vi "Fetch Waveform.vi"(8 "error in (no error)":errorcluster, 10 "Channel":string, 11 "Thermometer DAQmx Base CFG in":refnum<class "Thermometer DAQmx Base CFG.lvclass">) -> (0 "error out":errorcluster, 2 "Waveform":waveform(dbl), 3 "Thermometer DAQmx Base CFG out":refnum<class "Thermometer DAQmx Base CFG.lvclass">)   [LabVIEW 2023, in "Thermometer DAQmx Base CFG.lvclass"]
uses:
  Thermometer DAQmx Base CFG.lvclass
  DAQmx/DAQmx Base CFG/DAQmx Base CFG.lvclass/DAQmx Base CFG.ctl
  Thermometer DAQmx Base CFG.lvclass/Thermometer DAQmx Base CFG.ctl
  <vilib>/DAQmx/read.llb/DAQmx Read (Analog 1D Wfm NChan NSamp).vi
  <vilib>/Waveform/WDTOps.llb/WDT Append Waveforms DBL.vi
  <vilib>/DAQmx/miscellaneous.llb/DAQmx Fill In Error Info.vi
  <vilib>/Utility/error.llb/Error Cluster From Error Code.vi
  <vilib>/ErrorRing/Error Ring.xnode
  <resource>/objmgr/daqmx.rc
  DAQmx/DAQmx Base CFG/DAQmx Base CFG.lvclass
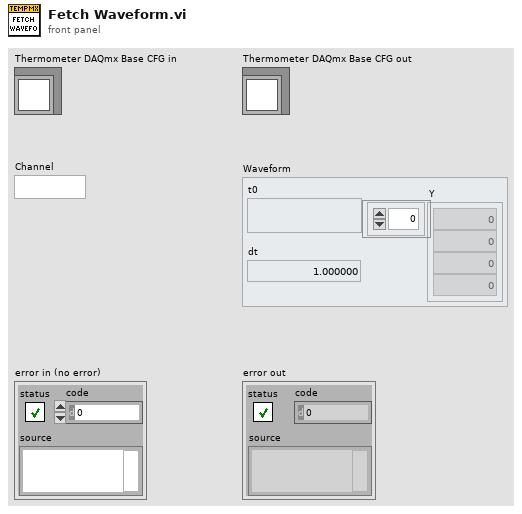
[diagram p1: front panel]
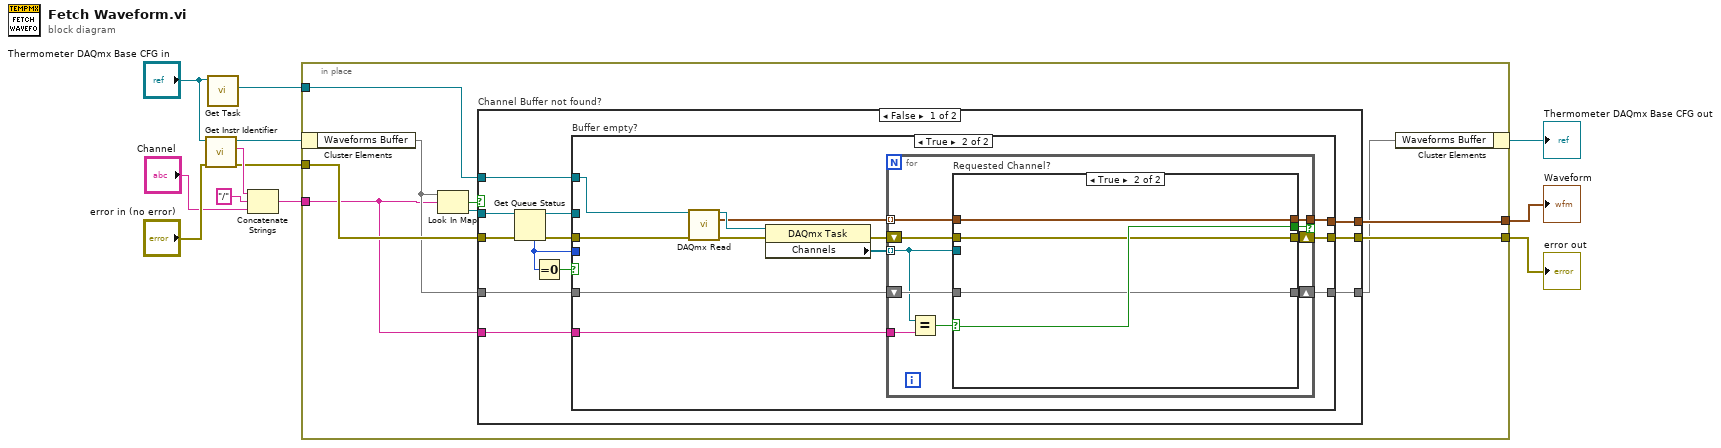
[diagram p0: block diagram]
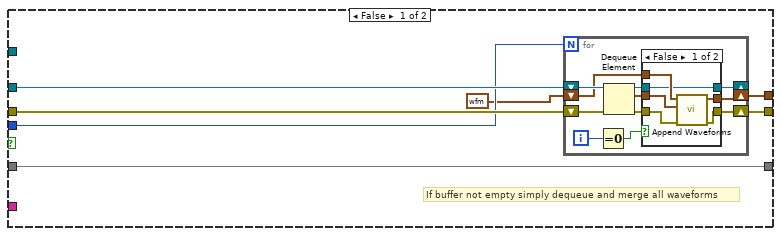
[diagram p2: hidden frame]
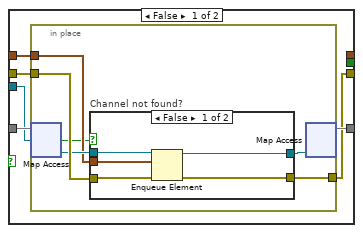
[diagram p4: hidden frame]
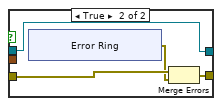
[diagram p5: hidden frame]
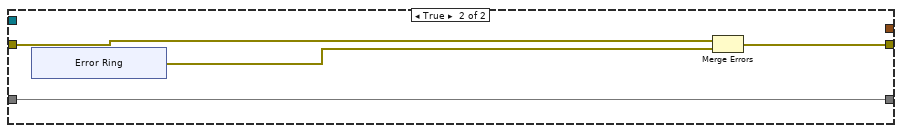
[diagram p6: hidden frame]
diagram:
  n1 = call-dynamic "Get Instr Identifier.vi"("error in (no error)"="error in (no error)", "Configuration Base in"="Thermometer DAQmx Base CFG in") -> ("error out"=w6:errorcluster, "Instr Ident"=w11:string, "Configuration Base out"=w8:refnum<class "Thermometer DAQmx Base CFG.lvclass">)  [unwired: 7 in]
  n2 = call "Get Task.vi"("DAQmx Base CFG in"="Thermometer DAQmx Base CFG in") -> ("Task"=w1:refnum<k21>)  [unwired: 9 in, 1 out]
  n3 = Concatenate Strings(w11, "/" ("string"), "Channel") -> (w7:string)
  n4 = in-place {
    in-place-border: w7 -> [w17]
    in-place-border: w6 -> [w21]
    in-place-border: [w20] -> w5
    in-place-border: [w19] -> w4
    in-place-border: w1 -> [w13]
    n5 = in-place-cluster #1(w8) -> ("Waveforms Buffer"=w18:map{string, refnum<queue>})
    n6 = Look In Map(map=w18, key=w17) -> (key not found?=w16:bool, value=w15:refnum<queue>)  [unwired: 1 in]
    n7 = case "Channel Buffer not found?" shown="False" w16 {
      tunnel: w21 -> [w33 w116]
      tunnel: [w31 w115] -> w19
      tunnel: [w29 _] -> w20
      tunnel: w13 -> [w26 _]
      tunnel: w15 -> [w27 _]
      tunnel: w17 -> [w25 _]
      tunnel: w18 -> [w24 w113]
      tunnel: [w22 w113] -> w14
      frame False {
        n8 = Get Queue Status(queue=w27, error in (no error)=w33) -> (queue out=w30:refnum<queue>, error out=w32:errorcluster, # elements in queue=w23:i32)  [unwired: 1 in, 5 out]
        n9 = Equal To 0?(x=w23) -> (x = 0?=w28:bool)
        n10 = case "Buffer empty?" shown="True" w28 {
          tunnel: w32 -> [w40 w72]
          tunnel: [w39 w63] -> w31
          tunnel: w30 -> [w38 _]
          tunnel: [w37 w64] -> w29
          tunnel: w26 -> [_ w61]
          tunnel: w25 -> [_ w66]
          tunnel: w24 -> [w34 w67]
          tunnel: w23 -> [w36 _]
          tunnel: [w34 w65] -> w22
          frame False {
            # "If buffer not empty simply dequeue and merge all waveforms"
            n11 = for {
              N: w36 -> [_]
              shift-right: [w48] -> w39
              shift-left: w40 -> [w51]
              shift-right: [w41] -> _
              shift-left: w38 -> [w49]
              shift-right: [w45] -> w37
              shift-left: waveform(dbl) {"t0"=timestamp(0 s since 1904-01-01), "dt"=1.0, "Y"=[]} ("Waveform") -> [w46]
              i -> [w44]
              n12 = Equal To 0?(x=w44) -> (x = 0?=w43:bool)
              n13 = Dequeue Element(queue=w49, error in (no error)=w51) -> (queue out=w42:refnum<queue>, element=w47:waveform(dbl), error out=w50:errorcluster)  [unwired: 1 in, 1 out]
              n14 = case shown="False" w43 {
                tunnel: w50 -> [w57 w58]
                tunnel: [w56 w58] -> w48
                tunnel: w47 -> [w55 w59]
                tunnel: w46 -> [w54 _]
                tunnel: [w53 w59] -> w45
                tunnel: w42 -> [w52 w60]
                tunnel: [w52 w60] -> w41
                frame False {
                  n15 = call-poly <vilib>:"Append Waveforms.vi"("error in (no error)"=w57, "waveform B"=w55, "waveform A"=w54) -> ("error out"=w56:errorcluster, "waveform out"=w53:waveform(dbl))  [unwired: 7 in]
                }
                frame True {
                }
              }
            }
          }
          frame True {
            n16 = call-poly <vilib>:"DAQmx Read.vi"("task/channels in"=w61, "error in"=w72) -> ("task out"=w70:refnum<k21>, "data"=w68:waveform(dbl)[], "error out"=w71:errorcluster)  [unwired: 11 in]
            n17 = property class="DAQmx Task"(reference=w70, error in=w71) -> (error out=w62:errorcluster, "Channels"=w69:refnum<k21>[])  [unwired: 1 out]
            n18 = for {
              tunnel: w69 -> [w74] mode=indexing
              tunnel: w68 -> [w81] mode=indexing
              tunnel: w66 -> [w80]
              shift-right: [w78] -> w65
              shift-left: w67 -> [w82]
              tunnel: [w77] -> w64 if=w76
              shift-right: [w75] -> w63
              shift-left: w62 -> [w73]
              n19 = Equal?(x=w74, y=w80) -> (x = y?=w79:bool)
              n20 = case "Requested Channel?" shown="True" w79 {
                selector: w79 -> [_ w111]
                tunnel: w82 -> [w88 w110]
                tunnel: w74 -> [w87 _]
                tunnel: w73 -> [w86 w109]
                tunnel: w81 -> [w85 w112]
                tunnel: [w84 w110] -> w78
                tunnel: [_ w112] -> w77
                tunnel: [_ w111] -> w76
                tunnel: [w83 w109] -> w75
                frame False {
                  n21 = in-place {
                    in-place-border: w86 -> [w94]
                    in-place-border: w85 -> [w92]
                    in-place-border: [w89] -> w83
                    n22 = in-place-map #2(w88, w87) -> (w93:refnum<queue>, w91:bool)  [unwired: 1 in]
                    n23 = case "Channel not found?" shown="False" w91 {
                      tunnel: w94 -> [w99 w103]
                      tunnel: w93 -> [w98 w100]
                      tunnel: w92 -> [w97 _]
                      tunnel: [w95 w102] -> w89
                      tunnel: [w96 w100] -> w90
                      frame False {
                        n24 = Enqueue Element(queue=w98, element=w97, error in (no error)=w99) -> (queue out=w96:refnum<queue>, error out=w95:errorcluster)  [unwired: 1 in, 1 out]
                      }
                      frame True {
                        n25 = xnode "Error Ring"() -> ("error out"=w101:errorcluster)
                        n26 = Merge Errors(w103, w101) -> (w102:errorcluster)
                      }
                    }
                    n27 = in-place-map #2(w90) -> (w84:map{string, refnum<queue>})  [unwired: 1 in, 2 out]
                  }
                }
                frame True {
                }
              }
            }
          }
        }
      }
      frame True {
        n28 = xnode "Error Ring"() -> ("error out"=w114:errorcluster)
        n29 = Merge Errors(w116, w114) -> (w115:errorcluster)
      }
    }
    n30 = in-place-cluster #1("Waveforms Buffer"=w14) -> (→"Thermometer DAQmx Base CFG out":refnum<class "Thermometer DAQmx Base CFG.lvclass">)
  }
  "error out" <- w4
  "Waveform" <- w5
